vi "Config AO Wav.vi"(6 "Channel config":T1={"Frequency"=10.0, "Voltage"=1.0, "Signal type"=enum."Sine Wave", "Square wave duty cycle (%)"=50.0, "physical channels"="", "name to assign"=""} {"Square wave duty cycle (%)" format="%0.2f"}, 7 "Sampling info":cluster{"Fs":dbl, "#s":dbl}={"Fs"=1000.0, "#s"=1000.0} {"Fs" format="%.2p"}, 8 "error in":errorcluster, 11 "task in":refnum<k21>) -> (0 "error out":errorcluster, 3 "task out":refnum<k21>, 4 "AO Waveform Graph":waveform(dbl)(graph))   [LabVIEW 2019]
doc: "This example demonstrates how to acquire a continuous amount of data (Waveform) using the DAQ device's internal clock. It also shows how to synchronize two devices for different device families (E Series, S Series, M Series, X Series, DSA, and SC Express), to simultaneously acquire the data.\n\nFor instructions on how to connect your signals to the DAQ device, refer to your device documentation."
uses:
  <vilib>/DAQmx/write.llb/DAQmx Write (Analog Wfm 1Chan NSamp).vi
  <vilib>/DAQmx/create/channels.llb/DAQmx Create Channel (AO-Voltage-Basic).vi
  <vilib>/DAQmx/configure/timing.llb/DAQmx Timing (Sample Clock).vi
  <vilib>/DAQmx/miscellaneous.llb/DAQmx Fill In Error Info.vi
  <vilib>/measure/NI_MABase.lvlib
panel:
  # "Config AO - Waveform"
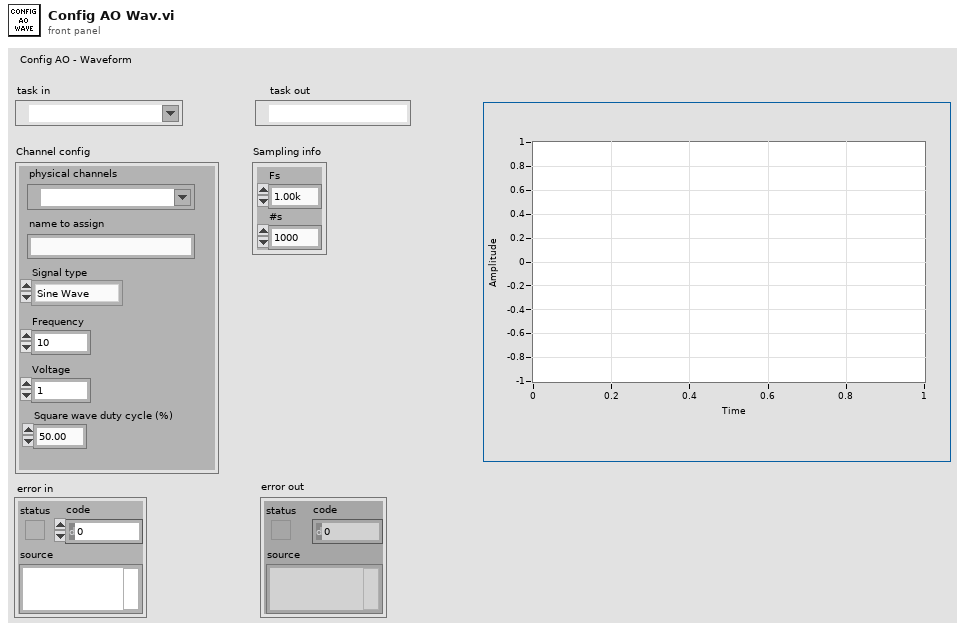
[diagram p1: front panel]
types:
  T1 = cluster{"Frequency":dbl, "Voltage":dbl, "Signal type":enum16{"Sine Wave", "Triangle Wave", "Square Wave", "Sawtooth Wave"}, "Square wave duty cycle (%)":dbl, "physical channels":tag, "name to assign":string}
  T2 = enum16{"Sine Wave", "Triangle Wave", "Square Wave", "Sawtooth Wave"}
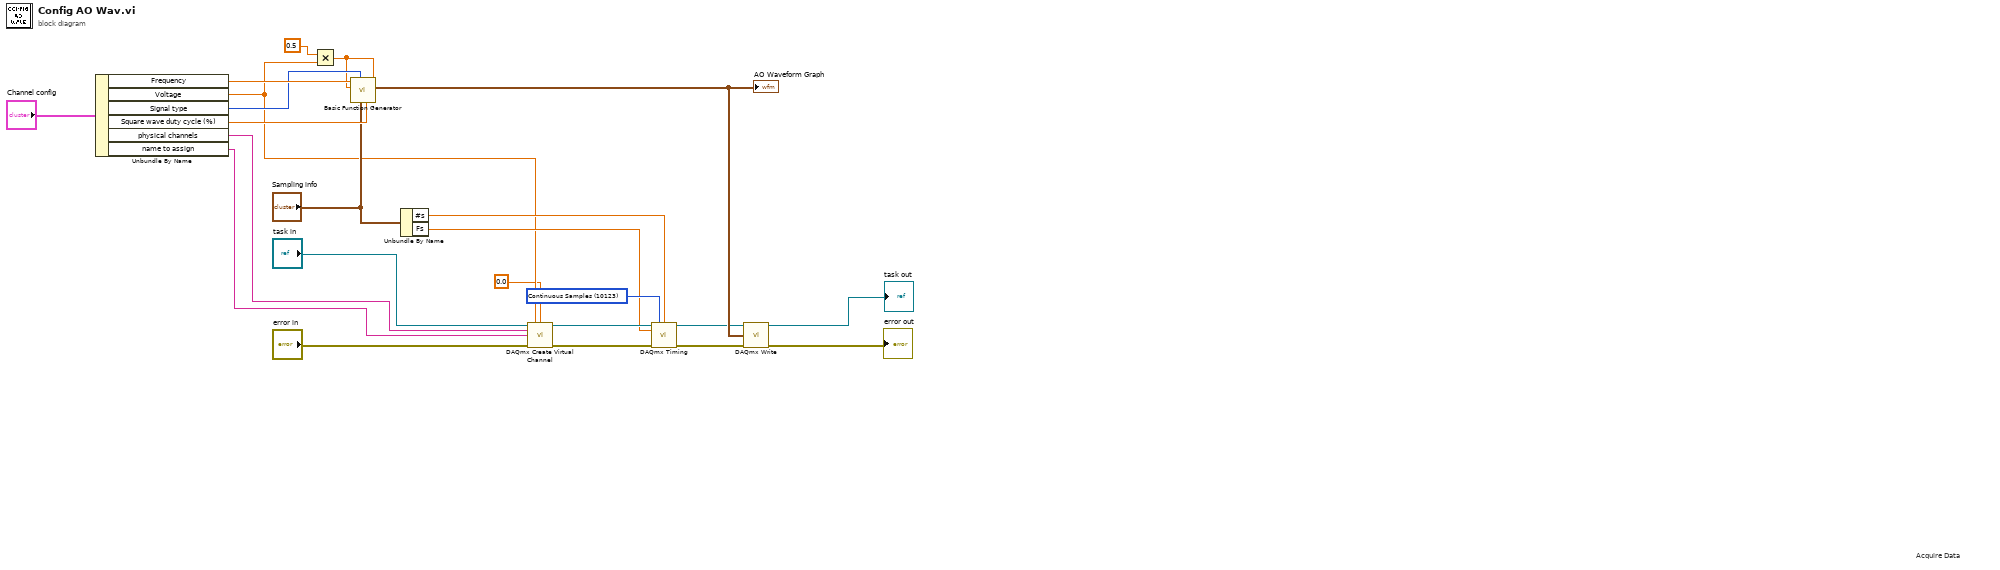
[diagram p0: block diagram]
diagram:
  w9 = 10123 items=["Finite Samples"=10178, "Continuous Samples"=10123, "Hardware Timed Single Point"=12522] ("sample mode")
  # "Acquire Data"
  n1 = Unbundle By Name("Channel config") -> ("Frequency"=w17:dbl, "Voltage"=w4:dbl, "Signal type"=w15:T2, "Square wave duty cycle (%)"=w16:dbl, "physical channels"=w2:tag, "name to assign"=w1:string)
  n2 = Multiply(x=0.5, y=w4) -> (x*y=w5:dbl)
  n3 = call <vilib>:"Basic Function Generator.vi"("offset"=w5, "square wave duty cycle (%)"=w16, "sampling info"="Sampling info", "signal type"=w15, "amplitude"=w5, "frequency"=w17) -> ("signal out"=w23:waveform(dbl))  [unwired: 3 in, 2 out]
  "AO Waveform Graph" <- w23
  n4 = Unbundle By Name("Sampling info") -> ("#s"=w8:dbl, "Fs"=w7:dbl)
  n5 = call-poly <vilib>:"DAQmx Create Virtual Channel.vi"("task in"="task in", "maximum value"=w4, "minimum value"=0.0, "physical channels"=w2, "name to assign"=w1, "error in"="error in") -> ("task out"=w14:refnum<k21>, "error out"=w13:errorcluster)  [unwired: 8 in]
  n6 = call-poly <vilib>:"DAQmx Timing.vi"("task/channels in"=w14, "sample mode"=w9, "samples per channel"=w8, "rate"=w7, "error in"=w13) -> ("task out"=w11:refnum<k21>, "error out"=w12:errorcluster)  [unwired: 9 in]
  n7 = call-poly <vilib>:"DAQmx Write.vi"("task/channels in"=w11, "data"=w23, "error in"=w12) -> ("task out"=→"task out":refnum<k21>, "error out"=→"error out":errorcluster)  [unwired: 10 in, 1 out]
